vi "Get to lower angle.vi"(2 "error in (no error)":errorcluster) -> (0 "error out":errorcluster)   [LabVIEW 2013]
uses:
  InTake Global Data.vi
  Cannon/Cannon Global Data.vi
panel:
  in  "wanted angle intake":dbl format="%#_13g"
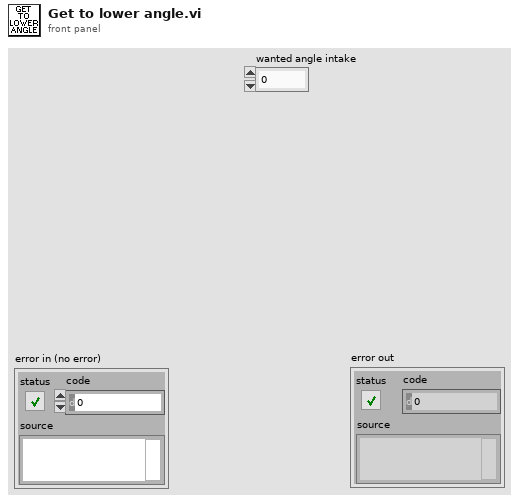
[diagram p1: front panel]
types:
  T1 = cluster{"TakeBall":dbl, "UpperClaw":dbl, "MS":bool, "Upper claw max":bool, "Upper claw min":bool, "Angle":dbl}
  T2 = typedef "WPI_SolenoidValue.ctl" = enum16{"Off", "On", "Forward", "Reverse"}
  T3 = cluster{"MS":bool, "Shoot!":T2, "Angle":dbl, "Lower claw max":bool, "Lower claw min":bool, "LowerClaw":dbl}
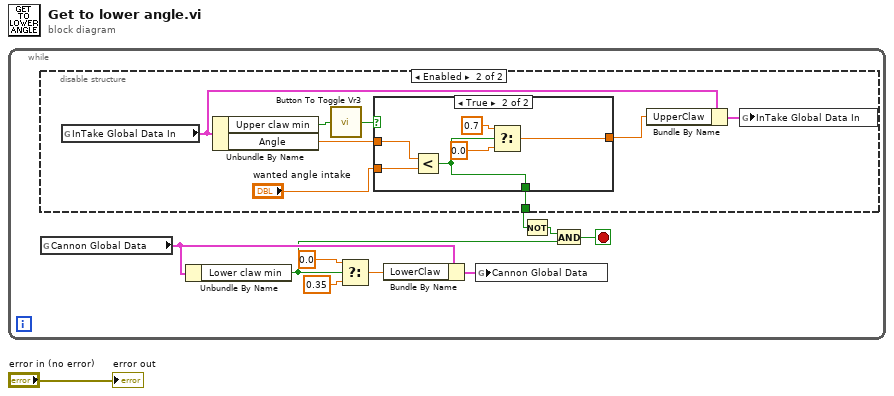
[diagram p0: block diagram]
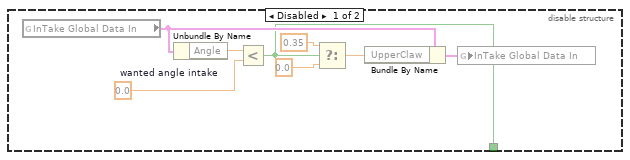
[diagram p2: hidden frame]
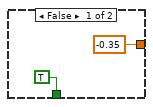
[diagram p3: hidden frame]
diagram:
  n1 = while {
    stop <- w6 stop-if-true
    n2 = disable-structure shown="Enabled" {
      disable-tunnel: [w11 w19] -> w10
      frame Disabled {
        w15 = 0.0  # wanted angle intake
        n3 = global read "InTake Global Data.vi" "InTake Global Data In"() -> (w17:T1)
        n4 = Unbundle By Name(w17) -> ("Angle"=w16:dbl)
        n5 = Less?(x=w16, y=w15) -> (x < y?=w11:bool)
        n6 = Select(t=0.35, s=w11, f=0.0) -> (s? t:f=w12:dbl)
        n7 = Bundle By Name(cluster=w17, "UpperClaw"=w12) -> (w18:T1)
        n8 = global write "InTake Global Data.vi" "InTake Global Data In"(w18) -> ()
      }
      frame Enabled {
        n9 = global read "InTake Global Data.vi" "InTake Global Data In"() -> (w26:T1)
        n10 = Unbundle By Name(w26) -> ("Upper claw min"=w21:bool, "Angle"=w22:dbl)
        n11 = call "Button To Toggle Vr3.vi"("InValue"=w21) -> ("Result"=w20:bool)
        n12 = case shown="True" w20 {
          tunnel: w22 -> [_ w34]
          tunnel: "wanted angle intake" -> [_ w33]
          tunnel: [-0.35 ("f") w30] -> w25
          tunnel: [TRUE w29] -> w19
          frame False {
          }
          frame True {
            n13 = Less?(x=w34, y=w33) -> (x < y?=w29:bool)
            n14 = Select(t=0.7, s=w29, f=0.0) -> (s? t:f=w30:dbl)
          }
        }
        n15 = Bundle By Name(cluster=w26, "UpperClaw"=w25) -> (w24:T1)
        n16 = global write "InTake Global Data.vi" "InTake Global Data In"(w24) -> ()
      }
    }
    n17 = global read "Cannon Global Data.vi" "Cannon Global Data"() -> (w3:T3)
    n18 = Unbundle By Name(w3) -> ("Lower claw min"=w2:bool)
    n19 = Select(t=0.0 ("f"), s=w2, f=0.35 ("t")) -> (s? t:f=w4:dbl)
    n20 = Bundle By Name(cluster=w3, "LowerClaw"=w4) -> (w5:T3)
    n21 = global write "Cannon Global Data.vi" "Cannon Global Data"(w5) -> ()
    n22 = Not(x=w10) -> (.not. x?=w9:bool)
    n23 = And(x=w9, y=w2) -> (x .and. y?=w6:bool)
  }
  "error out" <- "error in (no error)"
